vi "mqttCmdSubscribeSubInfoWrite.vi"(0 "mqttSubscribe in":refnum<class "mqttCmdSubscribe.lvclass">, 5 "subscriptionInfo":T1[](array[typedef])=[{"Topic"="a/b", "QoS"=enum."At least once"}], 11 "error in (no error)":errorcluster) -> (4 "mqttSubscribe out":refnum<class "mqttCmdSubscribe.lvclass">, 15 "error out":errorcluster)   [LabVIEW 2017, in "mqttCmdSubscribe.lvclass"]
uses:
  mqttCmdSubscribe.lvclass
  mqttTypedef/mqttSubscribeCluster.ctl
  mqttTypedef/mqttQOSlevel.ctl
  mqttCmdSubscribe.lvclass/mqttCmdSubscribe.ctl
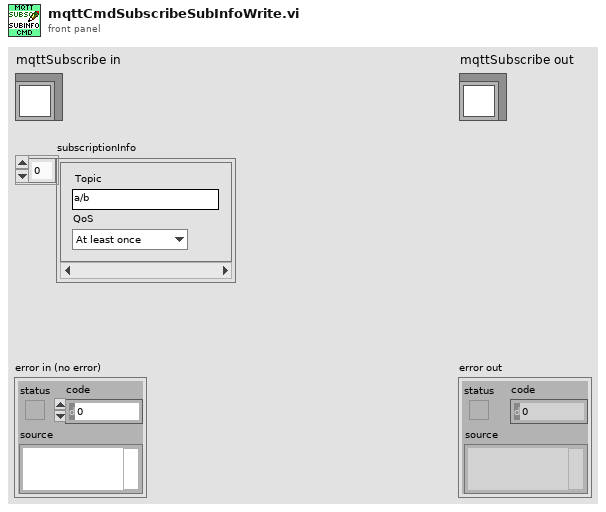
[diagram p1: front panel]
types:
  T1 = typedef "mqttSubscribeCluster.ctl" = cluster{"Topic":string, "QoS":T2}
  T2 = typedef "mqttQOSlevel.ctl" = enum8{"At most once", "At least once", "Exactly once", "Reserved"}
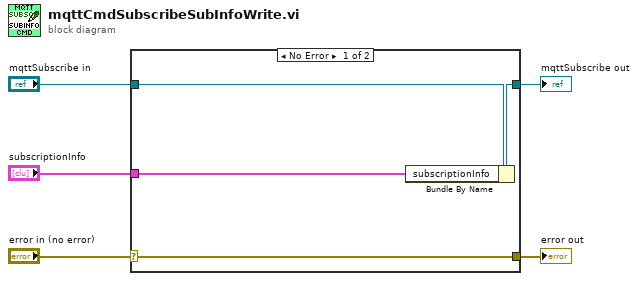
[diagram p0: block diagram]
diagram:
  n1 = case shown="No Error" "error in (no error)" {
    selector: "error in (no error)" -> [w9 w10]
    tunnel: [w9 w10] -> w4
    tunnel: [w7 w11] -> w2
    tunnel: "mqttSubscribe in" -> [w8 w11]
    tunnel: "subscriptionInfo" -> [w6 _]
    frame No Error {
      n2 = Bundle By Name(cluster=w8, "subscriptionInfo"=w6) -> (w7:refnum<class "mqttCmdSubscribe.lvclass">)
    }
    frame Error {
    }
  }
  "error out" <- w4
  "mqttSubscribe out" <- w2
